vi "Auto_Routine_LeftTwoPiece.vi"   [LabVIEW 2023]
uses:
  Arm2/ArmGetSetpointEnum.ctl
types:
  T1 = typedef "ArmGetSetpointEnum.ctl" = enum16{"ArmFloorPickup", "ArmAmpDeposit", "ArmSpeakerShoot", "ArmStartPosition", "ArmRestPosition", "ArmSourceIntake", "ArmAwayShoot"}
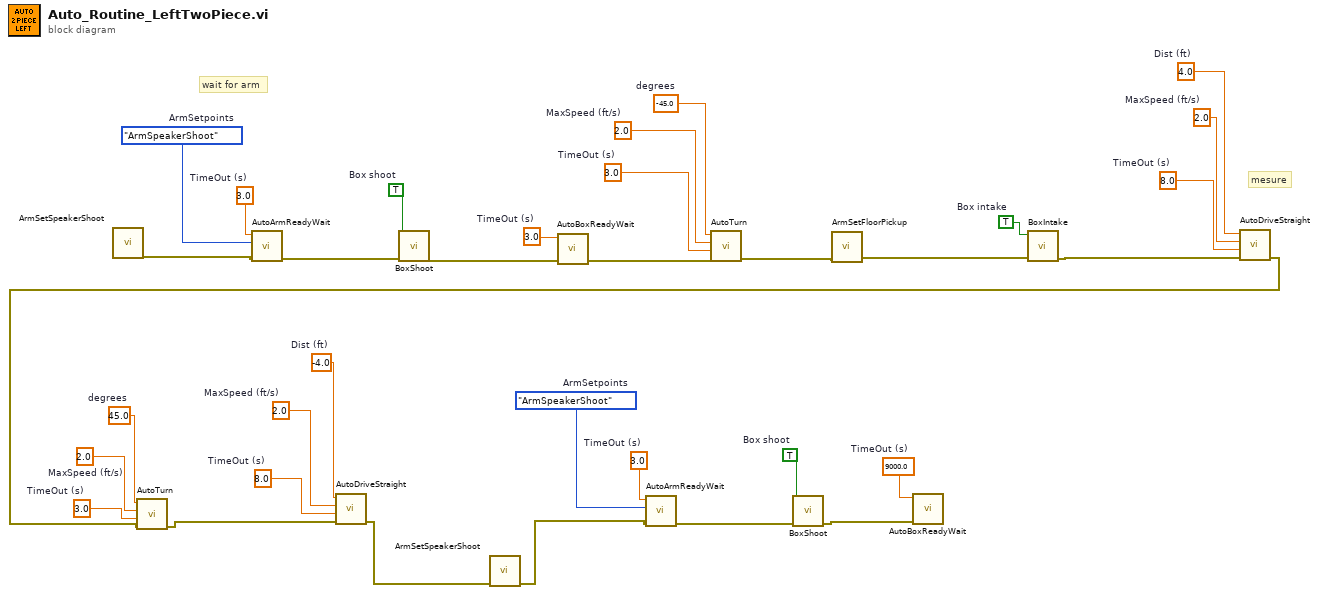
[diagram p0: block diagram]
diagram:
  w31 = 8.0  # TimeOut (s)
  w30 = 2.0  # MaxSpeed (ft/s)
  w29 = -4.0  # Dist (ft)
  w28 = 8.0  # TimeOut (s)
  w27 = 2.0  # MaxSpeed (ft/s)
  w26 = 4.0  # Dist (ft)
  w24 = 9000.0  # TimeOut (s)
  w23 = 3.0  # TimeOut (s)
  w22 = 2.0  # MaxSpeed (ft/s)
  w21 = 45.0  # degrees
  w20 = TRUE  # Box shoot
  w19 = ArmGetSetpointEnum."ArmSpeakerShoot"  # ArmSetpoints
  w18 = 3.0  # TimeOut (s)
  w15 = 3.0  # TimeOut (s)
  w14 = 2.0  # MaxSpeed (ft/s)
  w13 = -45.0  # degrees
  w10 = TRUE  # Box intake
  w9 = TRUE  # Box shoot
  w8 = ArmGetSetpointEnum."ArmSpeakerShoot"  # ArmSetpoints
  w7 = 3.0  # TimeOut (s)
  w1 = 3.0  # TimeOut (s)
  # "mesure"
  # "wait for arm"
  n1 = call "ArmSetSpeakerShoot.vi"() -> ("error out"=w2:errorcluster)  [unwired: 11 in]
  n2 = call "AutoArmReadyWait.vi"("error in (no error)"=w2, "ArmSetpoints"=w8, "TimeOut (s)"=w7) -> ("error out"=w3:errorcluster)  [unwired: 8 in]
  n3 = call "BoxShoot.vi"("error in (no error)"=w3, "Box shoot"=w9) -> ("error out"=w4:errorcluster)  [unwired: 9 in]
  n4 = call "AutoBoxReadyWait.vi"("error in (no error)"=w4, "TimeOut (s)"=w1) -> ("error out"=w11:errorcluster)  [unwired: 9 in]
  n5 = call "AutoTurn.vi"("error in (no error)"=w11, "TimeOut (s)"=w15, "MaxSpeed (ft/s)"=w14, "degrees"=w13) -> ("error out"=w12:errorcluster)  [unwired: 7 in]
  n6 = call "ArmSetFloorPickup.vi"("error in (no error)"=w12) -> ("error out"=w5:errorcluster)  [unwired: 10 in]
  n7 = call "BoxIntake.vi"("error in (no error)"=w5, "Box intake"=w10) -> ("error out"=w6:errorcluster)  [unwired: 9 in]
  n8 = call "AutoDriveStraight.vi"("error in (no error)"=w6, "TimeOut (s)"=w28, "MaxSpeed (ft/s)"=w27, "Dist (ft)"=w26) -> ("error out"=w34:errorcluster)  [unwired: 7 in]
  n9 = call "AutoTurn.vi"("error in (no error)"=w34, "TimeOut (s)"=w23, "MaxSpeed (ft/s)"=w22, "degrees"=w21) -> ("error out"=w33:errorcluster)  [unwired: 7 in]
  n10 = call "AutoDriveStraight.vi"("error in (no error)"=w33, "TimeOut (s)"=w31, "MaxSpeed (ft/s)"=w30, "Dist (ft)"=w29) -> ("error out"=w32:errorcluster)  [unwired: 7 in]
  n11 = call "ArmSetSpeakerShoot.vi"("error in (no error)"=w32) -> ("error out"=w16:errorcluster)  [unwired: 10 in]
  n12 = call "AutoArmReadyWait.vi"("error in (no error)"=w16, "ArmSetpoints"=w19, "TimeOut (s)"=w18) -> ("error out"=w17:errorcluster)  [unwired: 8 in]
  n13 = call "BoxShoot.vi"("error in (no error)"=w17, "Box shoot"=w20) -> ("error out"=w25:errorcluster)  [unwired: 9 in]
  n14 = call "AutoBoxReadyWait.vi"("error in (no error)"=w25, "TimeOut (s)"=w24) -> ()  [unwired: 9 in, 1 out]
